vi "WPI_CameraAttribute Cache.vi"(10 "Attribute Names":string[](array[string]), 11 "Camera Address In":string) -> (3 "Attribute Info":T2(array[cluster]))   [LabVIEW 2017]
doc: "Not currently used, but this VI caches information about camera attributes. This will only be needed if we discover that camera attribute reads are slow.\n\nThis software is licensed. Open the labview\\readme\\WPI Robotics Library Open Source License.txt file for more information."
uses:
  <vilib>/vision/driver/IMAQdx.llb/IMAQdx Attribute Type.ctl
  <vilib>/vision/driver/IMAQdx.llb/IMAQdx Attribute Visibility.ctl
  <vilib>/vision/driver/NI_Vision_Acquisition_Software.lvlib
  <resource>/objmgr/imaqdx.rc
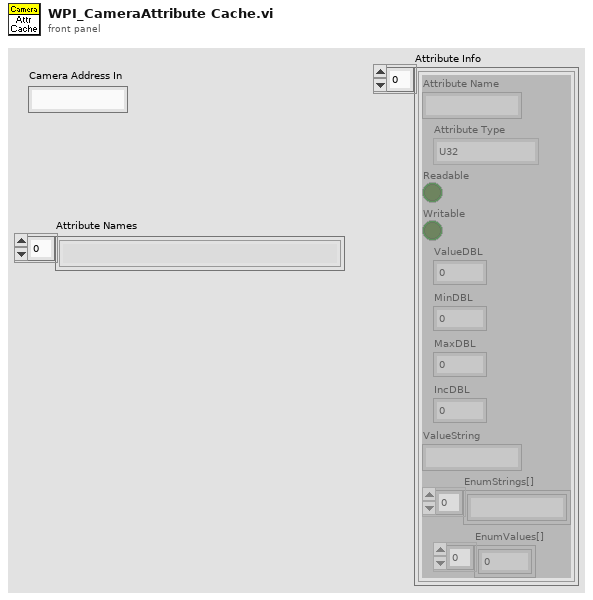
[diagram p1: front panel]
types:
  T1 = typedef "NI_Vision_Acquisition_Software.lvlib/IMAQdx Attribute Type.ctl" = enum32{"U32", "I64", "DBL", "String", "Enum", "Bool", "Command"}
  T2 = cluster{"Attribute Name":string, "Attribute Type":T1, "Readable":bool, "Writable":bool, "ValueDBL":dbl, "MinDBL":dbl, "MaxDBL":dbl, "IncDBL":dbl, "ValueString":string, "EnumStrings[]":string[], "EnumValues[]":u32[]}[]
  T3 = typedef "NI_Vision_Acquisition_Software.lvlib/IMAQdx Attribute Visibility.ctl" = enum32{"Simple", "Intermediate", "Advanced"}
  T4 = cluster{"Camera Address In":string, cluster{"Attribute Name":string, "Attribute Type":T1, "Readable":bool, "Writable":bool, "ValueDBL":dbl, "MinDBL":dbl, "MaxDBL":dbl, "IncDBL":dbl, "ValueString":string, "EnumStrings[]":string[], "EnumValues[]":u32[]}[]}[]
  T5 = cluster{"Attribute Type":T1, "Readable":bool, "Writable":bool, "Attribute Name":string}[]
  T6 = cluster{"Attribute Name":string, "Attribute Type":T1, "Readable":bool, "Writable":bool, "ValueDBL":dbl, "MinDBL":dbl, "MaxDBL":dbl, "IncDBL":dbl, "ValueString":string, "EnumStrings[]":string[], "EnumValues[]":u32[]}
  T7 = cluster{"Camera Address In":string, cluster{"Attribute Name":string, "Attribute Type":T1, "Readable":bool, "Writable":bool, "ValueDBL":dbl, "MinDBL":dbl, "MaxDBL":dbl, "IncDBL":dbl, "ValueString":string, "EnumStrings[]":string[], "EnumValues[]":u32[]}[]}
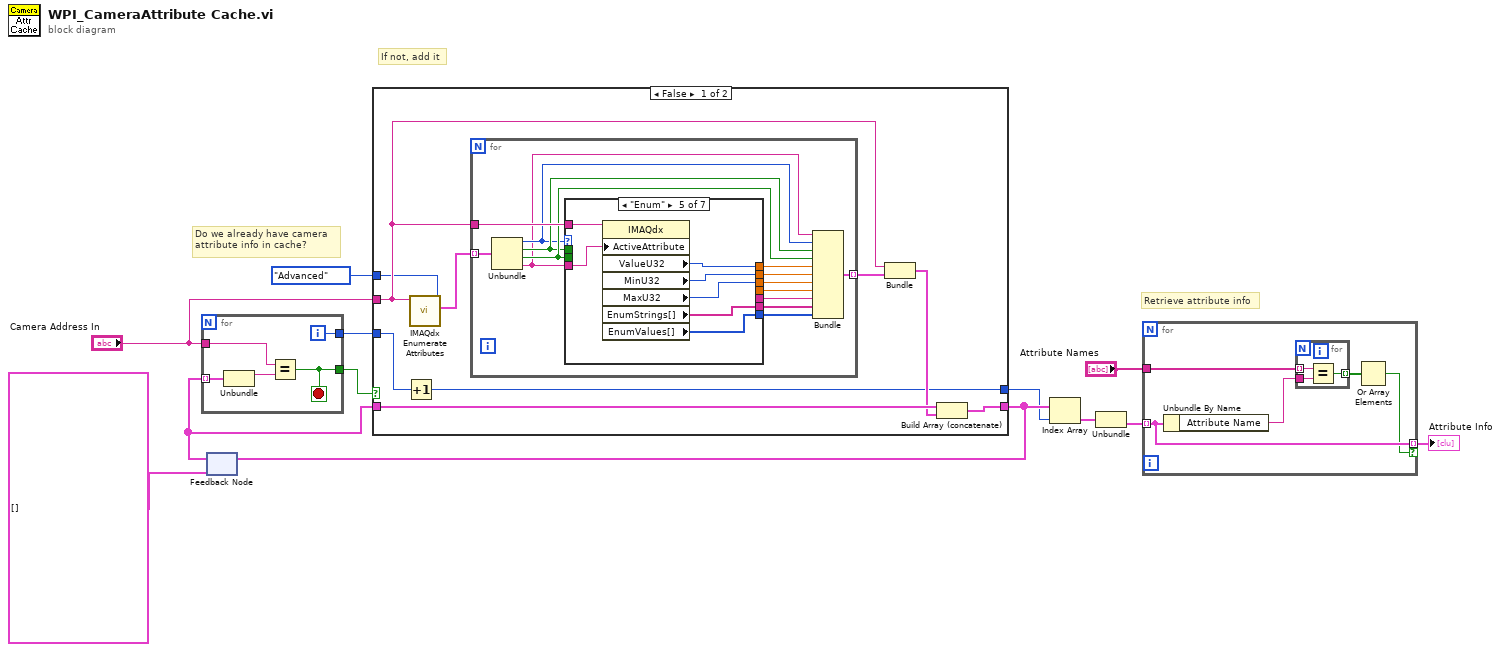
[diagram p0: block diagram]
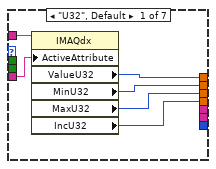
[diagram p2: hidden frame]
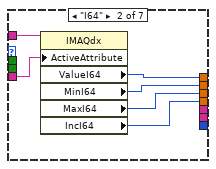
[diagram p3: hidden frame]
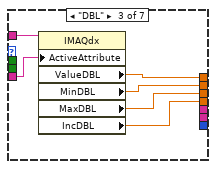
[diagram p4: hidden frame]
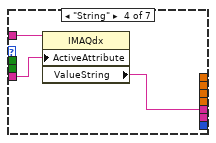
[diagram p5: hidden frame]
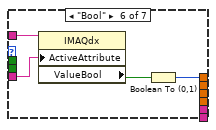
[diagram p6: hidden frame]
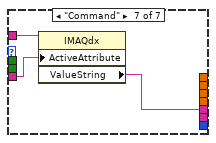
[diagram p7: hidden frame]
diagram:
  # "Retrieve attribute info"
  # "If not, add it"
  # "Do we already have camera\nattribute info in cache?"
  n1 = feedback #1(T4 []) -> (w9:T4)
  n2 = for {
    tunnel: "Camera Address In" -> [w16]
    tunnel: w9 -> [w15] mode=indexing
    tunnel: [w14] -> w11
    tunnel: [w13] -> w7
    i -> [w13]
    stop <- w14 stop-if-true
    n3 = Unbundle(w15) -> ("Camera Address In"=w17:string)  [unwired: 1 out]
    n4 = Equal?(x=w16, y=w17) -> (x = y?=w14:bool)
  }
  n5 = case shown="False" w11 {
    tunnel: "Camera Address In" -> [w23 _]
    tunnel: w9 -> [w26 w77]
    tunnel: [w25 w77] -> w6
    tunnel: IMAQdx_Attribute_Visibility."Advanced" ("Visibility") -> [w20 _]
    tunnel: w7 -> [w19 w76]
    tunnel: [w18 w76] -> w5
    frame False {
      n6 = Increment(x=w19) -> (x+1=w18:i32)
      n7 = call <vilib>:"IMAQdx Enumerate Attributes.vi"("Visibility"=w20, "Session In"=w23) -> ("Attribute Information Array"=w22:T5)  [unwired: 7 in, 2 out]
      n8 = for {
        tunnel: w22 -> [w40] mode=indexing
        tunnel: w23 -> [w39]
        tunnel: [w31] -> w24 mode=indexing
        n9 = Unbundle(w40) -> ("Attribute Type"=w28:T1, "Readable"=w29:bool, "Writable"=w30:bool, "Attribute Name"=w27:string)
        n10 = case shown="\"Enum\"" w28 {
          tunnel: w29 -> [_ _ _ _ _ _ _]
          tunnel: w30 -> [_ _ _ _ _ _ _]
          tunnel: w27 -> [w45 w52 w58 w60 w67 w71 w74]
          tunnel: w39 -> [w46 w51 w57 w61 w68 w72 w75]
          tunnel: [w44 w50 w56 _ w66 w69 _] -> w38
          tunnel: [w43 w49 w55 _ w65 _ _] -> w37
          tunnel: [w42 w48 w54 _ w64 _ _] -> w36
          tunnel: [w41 w47 w53 _ _ _ _] -> w35
          tunnel: [_ _ _ w59 _ _ w73] -> w34
          tunnel: [_ _ _ _ w62 _ _] -> w33
          tunnel: [_ _ _ _ w63 _ _] -> w32
          frame "U32", Default {
            n11 = property class="IMAQdx"(reference=w46, "ActiveAttribute"=w45) -> ("ValueU32"=w44:u32, "MinU32"=w43:u32, "MaxU32"=w42:u32, "IncU32"=w41:u32)  [unwired: 1 in, 2 out]
          }
          frame "I64" {
            n12 = property class="IMAQdx"(reference=w51, "ActiveAttribute"=w52) -> ("ValueI64"=w50:i64, "MinI64"=w49:i64, "MaxI64"=w48:i64, "IncI64"=w47:i64)  [unwired: 1 in, 2 out]
          }
          frame "DBL" {
            n13 = property class="IMAQdx"(reference=w57, "ActiveAttribute"=w58) -> ("ValueDBL"=w56:dbl, "MinDBL"=w55:dbl, "MaxDBL"=w54:dbl, "IncDBL"=w53:dbl)  [unwired: 1 in, 2 out]
          }
          frame "String" {
            n14 = property class="IMAQdx"(reference=w61, "ActiveAttribute"=w60) -> ("ValueString"=w59:string)  [unwired: 1 in, 2 out]
          }
          frame "Enum" {
            n15 = property class="IMAQdx"(reference=w68, "ActiveAttribute"=w67) -> ("ValueU32"=w66:u32, "MinU32"=w65:u32, "MaxU32"=w64:u32, "EnumStrings[]"=w63:string[], "EnumValues[]"=w62:u32[])  [unwired: 1 in, 2 out]
          }
          frame "Bool" {
            n16 = property class="IMAQdx"(reference=w72, "ActiveAttribute"=w71) -> ("ValueBool"=w70:bool)  [unwired: 1 in, 2 out]
            n17 = Boolean To (0,1)(Boolean=w70) -> (0, 1=w69:i16)
          }
          frame "Command" {
            n18 = property class="IMAQdx"(reference=w75, "ActiveAttribute"=w74) -> ("ValueString"=w73:string)  [unwired: 1 in, 2 out]
          }
        }
        n19 = Bundle("Attribute Name"=w27, "Attribute Type"=w28, "Readable"=w29, "Writable"=w30, "ValueDBL"=w38, "MinDBL"=w37, "MaxDBL"=w36, "IncDBL"=w35, "ValueString"=w34, "EnumStrings[]"=w32, "EnumValues[]"=w33) -> (w31:T6)  [unwired: 1 in]
      }
      n20 = Bundle("Camera Address In"=w23, w24) -> (w21:T7)  [unwired: 1 in]
      n21 = Build Array (concatenate)(w26, w21) -> (w25:T4)
    }
    frame True {
    }
  }
  n22 = feedback-in #1(w6) -> ()
  n23 = Index Array(array=w6, index=w5) -> (element=w4:T7)
  n24 = Unbundle(w4) -> (w3:T2)  [unwired: 1 out]
  n25 = for {
    tunnel: w3 -> [w79] mode=indexing
    tunnel: "Attribute Names" -> [w82]
    tunnel: [w79] -> w1 mode=indexing if=w78
    n26 = Unbundle By Name(w79) -> ("Attribute Name"=w80:string)
    n27 = for {
      tunnel: w80 -> [w85]
      tunnel: w82 -> [w84] mode=indexing
      tunnel: [w83] -> w81 mode=indexing
      n28 = Equal?(x=w84, y=w85) -> (x = y?=w83:bool)
    }
    n29 = Or Array Elements(Boolean array=w81) -> (logical OR=w78:bool)
  }
  "Attribute Info" <- w1
